vi "readFromXML.vi"(8 "error in (no error)":errorcluster, 10 "XML in":string, 11 "MccRotTrack in":refnum<class "MccRotTrack.lvclass">) -> (0 "error out":errorcluster, 3 "MccRotTrack out":refnum<class "MccRotTrack.lvclass">)   [LabVIEW 2022 SP3, in "TCSDataDefinitions.lvlib" / "TCSMountControlCommand.lvlib" / "CommandsForRotatorAxis.lvlib" / "MccRotTrack.lvclass"]
uses:
  MccRotTrack.lvclass
  Enumerations/MountTrackStates.ctl
  MccRotTrack.lvclass/MccRotTrack.ctl
  CommandsForRotatorAxis.lvclass
  <userlib>/Common/XML/XMLParser/XMLParser.lvclass
  TCSMountControlCommand.lvlib
panel:
  out "data":T1
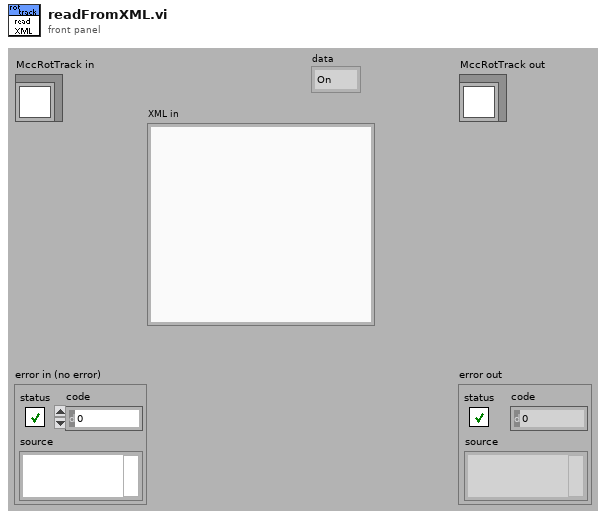
[diagram p1: front panel]
types:
  T1 = typedef "TCSDataDefinitions.lvlib/TCSMountControlCommand.lvlib/MountTrackStates.ctl" = enum16{"On", "Off"}
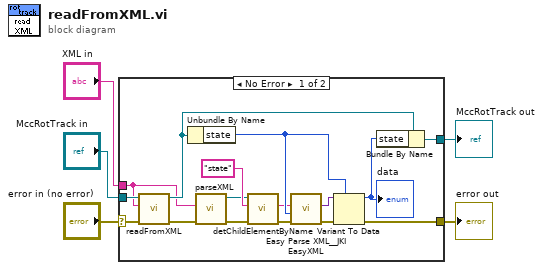
[diagram p0: block diagram]
diagram:
  n1 = case shown="No Error" "error in (no error)" {
    selector: "error in (no error)" -> [w17 w23]
    tunnel: [w16 w23] -> w4
    tunnel: [w13 w22] -> w2
    tunnel: "MccRotTrack in" -> [w19 w22]
    tunnel: "XML in" -> [w8 _]
    frame No Error {
      n2 = call-parent "readFromXML.vi"("error in (no error)"=w17, "XML in"=w8, "CommandsForRotatorAxis in"=w19) -> ("error out"=w12:errorcluster, "CommandsForRotatorAxis out"=w15:refnum<class "MccRotTrack.lvclass">)  [unwired: 7 out]
      n3 = Unbundle By Name(w15) -> ("state"=w18:T1)
      n4 = call <userlib>:"parseXML.vi"("error in (no error)"=w12, "XMLString in"=w8) -> ("error out"=w11:errorcluster, "Element out"=w6:refnum<class "XMLParser.lvclass">)  [unwired: 8 in]
      n5 = call <userlib>:"detChildElementByName.vi"("error in (no error)"=w11, "childName"="state" ("ChildName"), "Element in"=w6) -> ("error out"=w10:errorcluster, "childXML"=w7:string)  [unwired: 5 in, 2 out]
      n6 = call <vilib>:"Easy Parse XML__JKI EasyXML.vi"("error in (no error)"=w10, "LabVIEW Data (Type)"=w18, "XML String"=w7) -> ("error out"=w21:errorcluster, "LabVIEW Data"=w20:variant)  [unwired: 7 out]
      n7 = Variant To Data(error in=w21, type=w18, Variant=w20) -> (data=w14:T1, error out=w16:errorcluster)
      "data" <- w14
      n8 = Bundle By Name(cluster=w15, "state"=w14) -> (w13:refnum<class "MccRotTrack.lvclass">)
    }
    frame Error {
    }
  }
  "error out" <- w4
  "MccRotTrack out" <- w2
